vi "立体三体问题v1.vi"() -> ()   [LabVIEW 2018]
uses:
  <vilib>/gmath/NI_Gmath.lvlib
  <vilib>/Analysis/NI_AALBase.lvlib
  <vilib>/Native 3D Graph/xcontrol/3DPC_SurfacePlot.xctl
  <vilib>/Analysis/1siggen.llb/Ramp Pattern by Delta.vi
panel:
  in  "?":string[][](table)
  in  "半径":dbl=0.5
  in  "精度":dbl=1e-07 min=0.0 format="%#.15e"
  out "3D Graph":refnum<class "Base Datatype.lvclass">[](xcontrol)
  in  "m3":dbl=1.0 min=0.01
  in  "m2":dbl=1.0 min=0.01
  in  "m1":dbl=1.0 min=0.01
  in  "步长":dbl=0.0001 min=1e-20 format="%0.1e"
  in  "时间":dbl=10.0 min=0.0
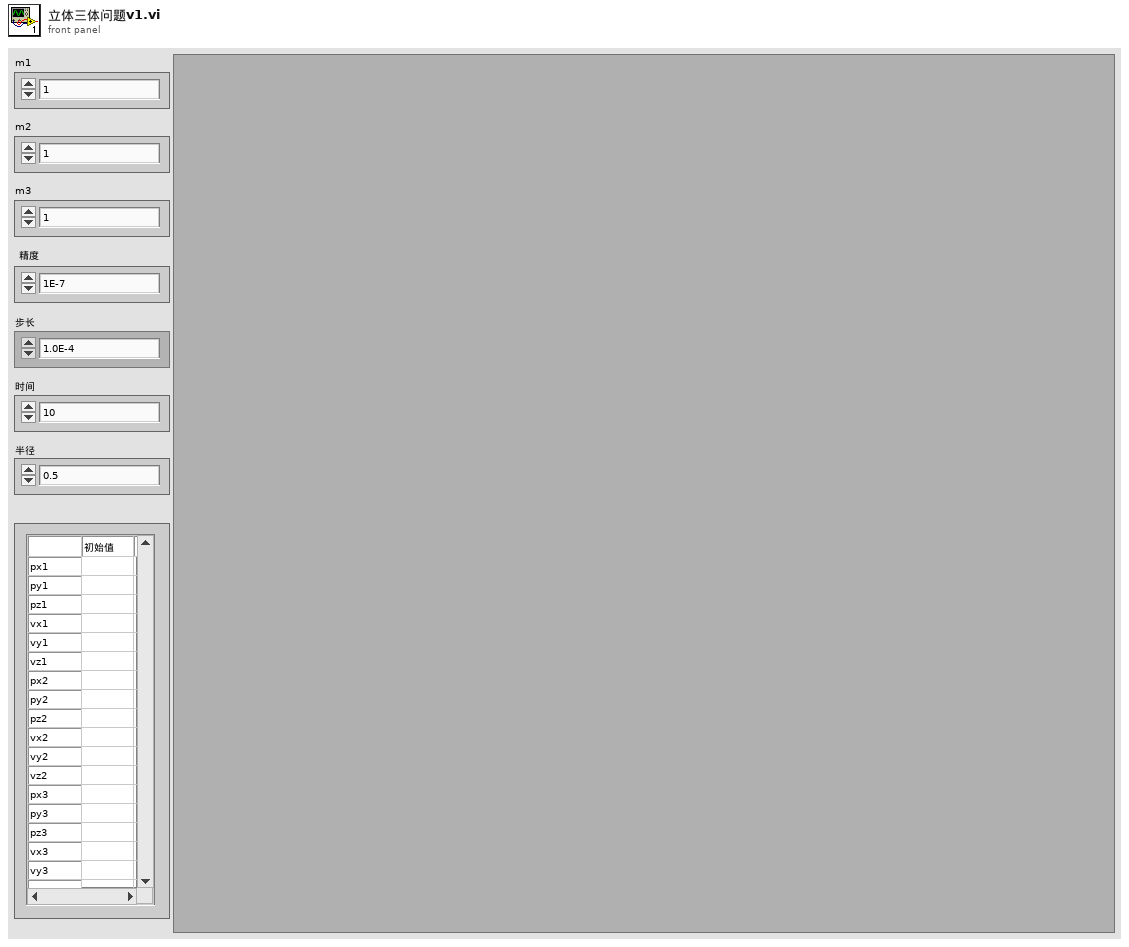
[diagram p1: front panel]
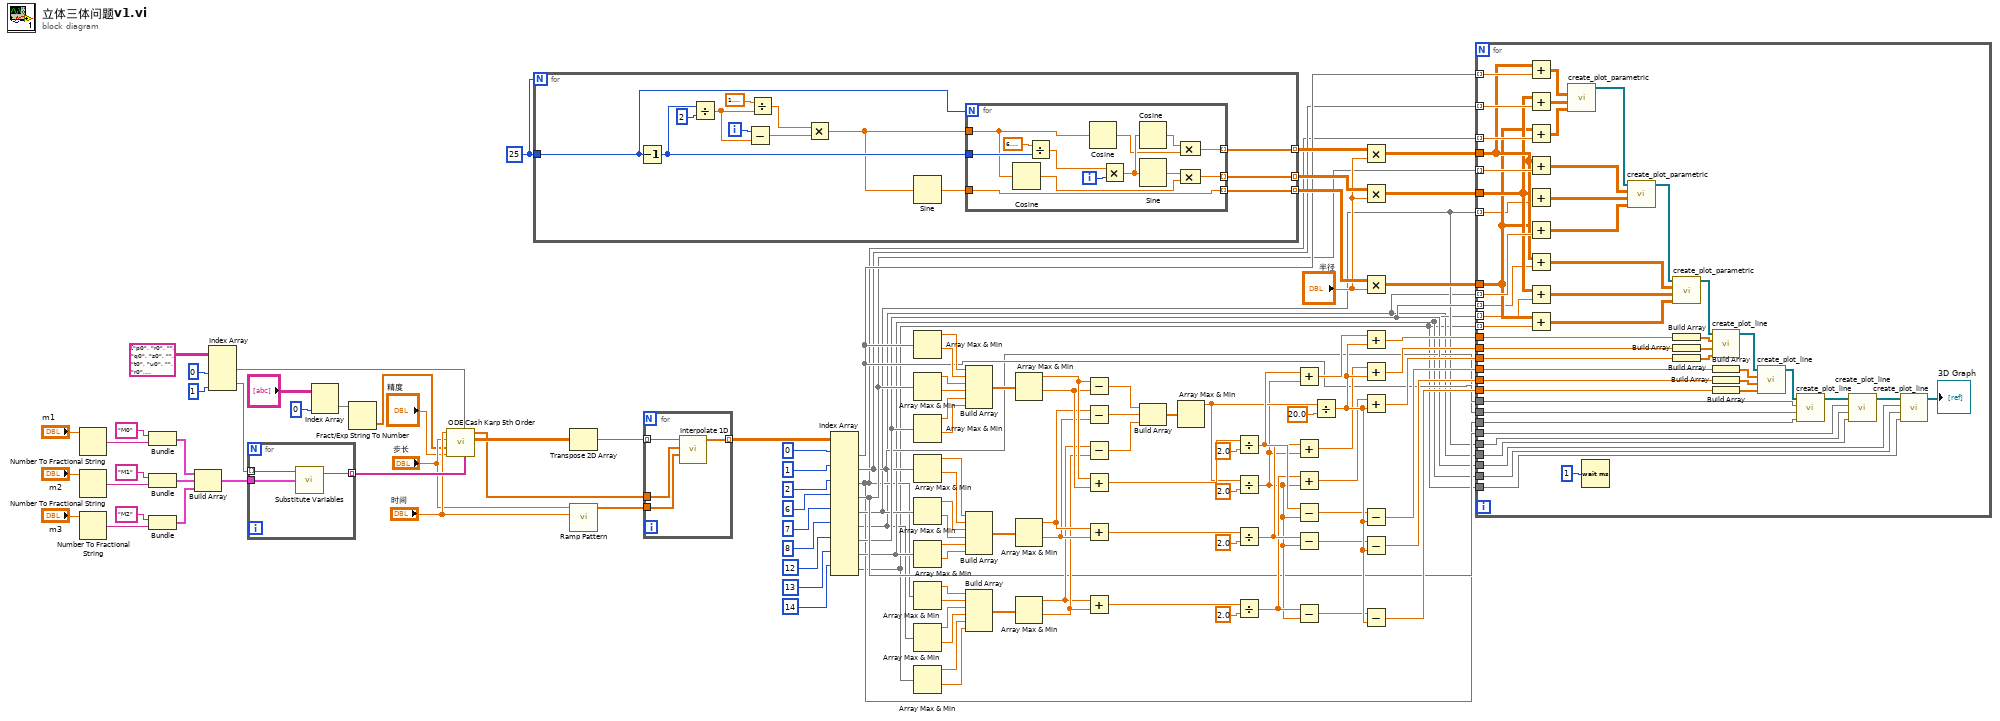
[diagram p0: block diagram]
diagram:
  w78 = 25
  n1 = Number To Fractional String(number="m1") -> (F-format string=w114:string)  [unwired: 3 out]
  n2 = Number To Fractional String(number="m2") -> (F-format string=w111:string)  [unwired: 3 out]
  n3 = Number To Fractional String(number="m3") -> (F-format string=w110:string)  [unwired: 3 out]
  n4 = Bundle("M0", w114) -> (w108:cluster{string, string})  [unwired: 1 out]
  n5 = Bundle("M1", w111) -> (w107:cluster{string, string})  [unwired: 1 out]
  n6 = Bundle("M2", w110) -> (w106:cluster{string, string})  [unwired: 1 out]
  n7 = Build Array(w108, w107, w106) -> (w105:cluster{string, string}[])
  n8 = Index Array(array=string[][] [["p0", "r0", ""], ["q0", "s0", ""], ["t0", "u0", ""], ["r0", "M1*(p1-p0)/sqrt((p1-p0)^2+(q1-q0)^2+(t1-t0)^2)^3+M2*(p2-p0)/sqrt((p2-p0)^2+(q2-q0)^2+(t1-t0)^2)^3", ""], ["s0", "M1*(q1-q0)/sqrt((p1-p0)^2+(q1-q0)^2+(t1-t0)^2)^3+M2*(q2-q0)/sqrt((p2-p0)^2+(q2-q0)^2+(t1-t0)^2)^3", ""], ["u0", "M1*(t1-t0)/sqrt((p1-p0)^2+(q1-q0)^2+(t1-t0)^2)^3+M2*(t2-t0)/sqrt((p2-p0)^2+(q2-q0)^2+(t1-t0)^2)^3", ""], ["p1", "r1", ""], ["q1", "s1", ""], ["t1", "u1", ""], ["r1", "M2*(p2-p1)/sqrt((p2-p1)^2+(q2-q1)^2+(t2-t1)^2)^3+M0*(p0-p1)/sqrt((p0-p1)^2+(q0-q1)^2+(t2-t1)^2)^3", ""], ["s1", "M2*(q2-q1)/sqrt((p2-p1)^2+(q2-q1)^2+(t2-t1)^2)^3+M0*(q0-q1)/sqrt((p0-p1)^2+(q0-q1)^2+(t2-t1)^2)^3", ""], ["u1", "M2*(t2-t1)/sqrt((p2-p1)^2+(q2-q1)^2+(t2-t1)^2)^3+M0*(t0-t1)/sqrt((p0-p1)^2+(q0-q1)^2+(t2-t1)^2)^3", ""], ["p2", "r2", ""], ["q2", "s2", ""], ["t2", "u2", ""], ["r2", "M0*(p0-p2)/sqrt((p0-p2)^2+(q0-q2)^2+(t0-t2)^2)^3+M1*(p1-p2)/sqrt((p1-p2)^2+(q1-q2)^2+(t0-t2)^2)^3", ""], ["s2", "M0*(q0-q2)/sqrt((p0-p2)^2+(q0-q2)^2+(t0-t2)^2)^3+M1*(q1-q2)/sqrt((p1-p2)^2+(q1-q2)^2+(t0-t2)^2)^3", ""], ["u2", "M0*(t0-t2)/sqrt((p0-p2)^2+(q0-q2)^2+(t0-t2)^2)^3+M1*(t1-t2)/sqrt((p1-p2)^2+(q1-q2)^2+(t0-t2)^2)^3", ""]] ("表格"), index (col) #1=0 ("disabled index (col)"), index (col) #2=1 ("index (col)")) -> (element #1=w92:string[], element #2=w93:string[])  [unwired: 2 in]
  n9 = for {
    tunnel: w93 -> [w118] mode=indexing
    tunnel: w105 -> [w116]
    tunnel: [w117] -> w115 mode=indexing
    n10 = call <vilib>:"Substitute Variables.vi"("Substitution Rules"=w116, "original formula"=w118) -> ("formula after substitution"=w117:string)  [unwired: 1 in, 1 out]
  }
  n11 = Index Array(array="?", index (col)=0 ("索引 (行)")) -> (element=w3:string[])  [unwired: 1 in]
  n12 = Fract/Exp String To Number(string=w3) -> (number=w90:dbl[])  [unwired: 3 in, 1 out]
  n13 = call <vilib>:"ODE Cash Karp 5th Order.vi"("F(X,t) (right sides of the ODE\nas functions of X and t)"=w115, "X (name of variables)"=w92, "accuracy"="精度", "X0"=w90, "h (step rate)"="步长", "time end"="时间") -> ("error"=w2:i32, "X Values (solution)"=w101:dbl[][], "Times"=w99:dbl[])  [unwired: 2 in, 1 out]
  n14 = for {
    N: w78 -> [_]
    tunnel: w78 -> [w131]
    tunnel: [w122] -> w76 mode=indexing
    tunnel: [w121] -> w74 mode=indexing
    tunnel: [w120] -> w72 mode=indexing
    i -> [w124]
    n15 = Decrement(x=w131) -> (x-1=w127:i32)
    n16 = Divide(x=w127, y=2) -> (x/y=w126:dbl)
    n17 = Subtract(x=w124, y=w126) -> (x-y=w129:dbl)
    n18 = Divide(x=1.5707963267948966, y=w126) -> (x/y=w130:dbl)
    n19 = Multiply(x=w130, y=w129) -> (x*y=w123:dbl)
    n20 = Sine(x=w123) -> (sin(x)=w119:dbl)
    n21 = for {
      N: w131 -> [_]
      tunnel: w127 -> [w143]
      tunnel: w123 -> [w139]
      tunnel: [w134] -> w122 mode=indexing
      tunnel: [w133] -> w121 mode=indexing
      tunnel: [w132] -> w120 mode=indexing
      tunnel: w119 -> [w132]
      i -> [w142]
      n22 = Cosine(x=w139) -> (cos(x)=w138:dbl)
      n23 = Divide(x=6.283185307179586, y=w143) -> (x/y=w141:dbl)
      n24 = Cosine(x=w139) -> (cos(x)=w136:dbl)
      n25 = Multiply(x=w141, y=w142) -> (x*y=w140:dbl)
      n26 = Cosine(x=w140) -> (cos(x)=w135:dbl)
      n27 = Sine(x=w140) -> (sin(x)=w137:dbl)
      n28 = Compound Arithmetic op=MULTIPLY(w135, w136) -> (w134:dbl)
      n29 = Compound Arithmetic op=MULTIPLY(w137, w138) -> (w133:dbl)
    }
  }
  n30 = Transpose 2D Array(2D array=w101) -> (transposed array=w98:dbl[][])
  n31 = call-poly <vilib>:"Ramp Pattern.vi"("end"="时间", "delta"="步长") -> ("Ramp Pattern"=w89:dbl[])  [unwired: 7 in, 2 out]
  n32 = for {
    tunnel: w98 -> [w148] mode=indexing
    tunnel: [w147] -> w100 mode=indexing
    tunnel: w99 -> [w146]
    tunnel: w89 -> [w145]
    n33 = call <vilib>:"Interpolate 1D.vi"("xi"=w145, "X"=w146, "Y"=w148) -> ("yi"=w147:dbl[])  [unwired: 6 in, 2 out]
  }
  n34 = Index Array(array=w100, index (row) #1=0 ("索引 (行)"), index (row) #2=1 ("索引 (行)"), index (row) #3=2 ("索引 (行)"), index (row) #4=6 ("索引 (行)"), index (row) #5=7 ("索引 (行)"), index (row) #6=8 ("索引 (行)"), index (row) #7=12 ("索引 (行)"), index (row) #8=13 ("索引 (行)"), index (row) #9=14 ("索引 (行)")) -> (element #1=w13:dbl[], element #2=w10:dbl[], element #3=w7:dbl[], element #4=w12:dbl[], element #5=w9:dbl[], element #6=w6:dbl[], element #7=w11:dbl[], element #8=w8:dbl[], element #9=w5:dbl[])  [unwired: 9 in]
  n35 = Array Max & Min(array=w13) -> (max value=w70:dbl, min value=w69:dbl)  [unwired: 2 out]
  n36 = Array Max & Min(array=w12) -> (max value=w68:dbl, min value=w67:dbl)  [unwired: 2 out]
  n37 = Array Max & Min(array=w11) -> (max value=w66:dbl, min value=w65:dbl)  [unwired: 2 out]
  n38 = Array Max & Min(array=w10) -> (max value=w64:dbl, min value=w63:dbl)  [unwired: 2 out]
  n39 = Array Max & Min(array=w9) -> (max value=w62:dbl, min value=w61:dbl)  [unwired: 2 out]
  n40 = Array Max & Min(array=w8) -> (max value=w60:dbl, min value=w59:dbl)  [unwired: 2 out]
  n41 = Array Max & Min(array=w7) -> (max value=w28:dbl, min value=w29:dbl)  [unwired: 2 out]
  n42 = Array Max & Min(array=w6) -> (max value=w30:dbl, min value=w31:dbl)  [unwired: 2 out]
  n43 = Array Max & Min(array=w5) -> (max value=w32:dbl, min value=w33:dbl)  [unwired: 2 out]
  n44 = Build Array(w70, w69, w68, w67, w66, w65) -> (w58:dbl[])
  n45 = Build Array(w64, w63, w62, w61, w60, w59) -> (w57:dbl[])
  n46 = Build Array(w28, w29, w30, w31, w32, w33) -> (w34:dbl[])
  n47 = Array Max & Min(array=w58) -> (max value=w50:dbl, min value=w49:dbl)  [unwired: 2 out]
  n48 = Array Max & Min(array=w57) -> (max value=w46:dbl, min value=w45:dbl)  [unwired: 2 out]
  n49 = Array Max & Min(array=w34) -> (max value=w35:dbl, min value=w36:dbl)  [unwired: 2 out]
  n50 = Subtract(x=w50, y=w49) -> (x-y=w56:dbl)
  n51 = Subtract(x=w46, y=w45) -> (x-y=w55:dbl)
  n52 = Subtract(x=w35, y=w36) -> (x-y=w27:dbl)
  n53 = Add(x=w50, y=w49) -> (x+y=w47:dbl)
  n54 = Add(x=w46, y=w45) -> (x+y=w43:dbl)
  n55 = Add(x=w35, y=w36) -> (x+y=w25:dbl)
  n56 = Build Array(w56, w55, w27) -> (w54:dbl[])
  n57 = Array Max & Min(array=w54) -> (max value=w23:dbl)  [unwired: 3 out]
  n58 = Divide(x=w47, y=2.0) -> (x/y=w41:dbl)
  n59 = Divide(x=w23, y=2.0) -> (x/y=w22:dbl)
  n60 = Divide(x=w43, y=2.0) -> (x/y=w38:dbl)
  n61 = Divide(x=w25, y=2.0) -> (x/y=w24:dbl)
  n62 = Add(x=w41, y=w22) -> (x+y=w42:dbl)
  n63 = Add(x=w38, y=w22) -> (x+y=w39:dbl)
  n64 = Add(x=w24, y=w22) -> (x+y=w21:dbl)
  n65 = Subtract(x=w41, y=w22) -> (x-y=w40:dbl)
  n66 = Subtract(x=w38, y=w22) -> (x-y=w37:dbl)
  n67 = Subtract(x=w24, y=w22) -> (x-y=w20:dbl)
  n68 = Divide(x=w23, y=20.0) -> (x/y=w53:dbl)
  n69 = Multiply(x=w76, y="半径") -> (x*y=w77:dbl[][])
  n70 = Multiply(x=w74, y="半径") -> (x*y=w75:dbl[][])
  n71 = Multiply(x=w72, y="半径") -> (x*y=w73:dbl[][])
  n72 = Add(x=w42, y=w53) -> (x+y=w19:dbl)
  n73 = Add(x=w39, y=w53) -> (x+y=w18:dbl)
  n74 = Add(x=w21, y=w53) -> (x+y=w17:dbl)
  n75 = Subtract(x=w40, y=w53) -> (x-y=w16:dbl)
  n76 = Subtract(x=w37, y=w53) -> (x-y=w15:dbl)
  n77 = Subtract(x=w20, y=w53) -> (x-y=w14:dbl)
  n78 = for {
    tunnel: w13 -> [w199] mode=indexing
    tunnel: w10 -> [w198] mode=indexing
    tunnel: w7 -> [w197] mode=indexing
    tunnel: w12 -> [w191] mode=indexing
    tunnel: w6 -> [w190] mode=indexing
    tunnel: w8 -> [w183] mode=indexing
    tunnel: w5 -> [w182] mode=indexing
    tunnel: w77 -> [w186]
    tunnel: w75 -> [w185]
    tunnel: w73 -> [w184]
    tunnel: w19 -> [w177]
    tunnel: w18 -> [w176]
    tunnel: w17 -> [w175]
    tunnel: w16 -> [w169]
    tunnel: w15 -> [w168]
    tunnel: w14 -> [w167]
    tunnel: w13 -> [w163]
    tunnel: w12 -> [w162]
    tunnel: w11 -> [w161]
    tunnel: w10 -> [w160]
    tunnel: w9 -> [w159]
    tunnel: w8 -> [w158]
    tunnel: w7 -> [w157]
    tunnel: w6 -> [w156]
    tunnel: w5 -> [w155]
    tunnel: w11 -> [w150] mode=indexing
    tunnel: w9 -> [w149] mode=indexing
    n79 = Add(x=w186, y=w199) -> (x+y=w178:dbl[][])
    n80 = Add(x=w185, y=w198) -> (x+y=w196:dbl[][])
    n81 = Add(x=w184, y=w197) -> (x+y=w195:dbl[][])
    n82 = Add(x=w186, y=w191) -> (x+y=w194:dbl[][])
    n83 = Add(x=w185, y=w149) -> (x+y=w193:dbl[][])
    n84 = Add(x=w184, y=w190) -> (x+y=w192:dbl[][])
    n85 = Add(x=w186, y=w150) -> (x+y=w187:dbl[][])
    n86 = Add(x=w185, y=w183) -> (x+y=w188:dbl[][])
    n87 = Add(x=w184, y=w182) -> (x+y=w189:dbl[][])
    n88 = call <vilib>:"create_plot_parametric.vi"("z matrix"=w195, "y matrix"=w196, "x matrix"=w178) -> ("plots out"=w181:refnum<class "Base Datatype.lvclass">[])  [unwired: 2 in, 6 out]
    n89 = Wait (ms)(milliseconds to wait=u32 1 ("等待时间（毫秒）")) -> ()  [unwired: 1 out]
    n90 = call <vilib>:"create_plot_parametric.vi"("z matrix"=w192, "y matrix"=w193, "x matrix"=w194, "plots in"=w181) -> ("plots out"=w180:refnum<class "Base Datatype.lvclass">[])  [unwired: 1 in, 6 out]
    n91 = call <vilib>:"create_plot_parametric.vi"("z matrix"=w189, "y matrix"=w188, "x matrix"=w187, "plots in"=w180) -> ("plots out"=w171:refnum<class "Base Datatype.lvclass">[])  [unwired: 1 in, 6 out]
    n92 = Build Array(w177) -> (w174:dbl[])
    n93 = Build Array(w176) -> (w173:dbl[])
    n94 = Build Array(w175) -> (w172:dbl[])
    n95 = call <vilib>:"create_plot_line.vi"("z vector"=w172, "y vector"=w173, "x vector"=w174, "plots in"=w171) -> ("plots out"=w170:refnum<class "Base Datatype.lvclass">[])  [unwired: 1 in, 6 out]
    n96 = Build Array(w169) -> (w166:dbl[])
    n97 = Build Array(w168) -> (w165:dbl[])
    n98 = Build Array(w167) -> (w164:dbl[])
    n99 = call <vilib>:"create_plot_line.vi"("z vector"=w164, "y vector"=w165, "x vector"=w166, "plots in"=w170) -> ("plots out"=w154:refnum<class "Base Datatype.lvclass">[])  [unwired: 1 in, 6 out]
    n100 = call <vilib>:"create_plot_line.vi"("z vector"=w157, "y vector"=w160, "x vector"=w163, "plots in"=w154) -> ("plots out"=w153:refnum<class "Base Datatype.lvclass">[])  [unwired: 1 in, 6 out]
    n101 = call <vilib>:"create_plot_line.vi"("z vector"=w156, "y vector"=w159, "x vector"=w162, "plots in"=w153) -> ("plots out"=w152:refnum<class "Base Datatype.lvclass">[])  [unwired: 1 in, 6 out]
    n102 = call <vilib>:"create_plot_line.vi"("z vector"=w155, "y vector"=w158, "x vector"=w161, "plots in"=w152) -> ("plots out"=→"3D Graph":refnum<class "Base Datatype.lvclass">[])  [unwired: 1 in, 6 out]
  }
